vi "Startup.vi"(8 "error in (no error)":errorcluster, 11 "MyApp in":refnum<class "MyApp.lvclass">) -> (0 "error out":errorcluster, 3 "MyApp out":refnum<class "MyApp.lvclass">)   [LabVIEW 2012, in "MyApp.lvlib" / "MyApp.lvclass"]
uses:
  MyApp.lvclass
  HGF_DataAnalyzer/Wfm_Amplitude/Wfm_Amplitude.lvclass
  HGF_DataAnalyzer/Wfm_PulseMeasurement/Wfm_PulseMeasurement.lvclass
  HGF_DataAnalyzer/WfmAnalysator/WfmAnalysator.lvclass
  HGF_LVC/HGF_ApplicationBaseClasses/HGF_Application/HGF_Application.lvclass
  MyApp.lvclass/MyApp.ctl
  HGF_LVC/HGF_BaseClasses/HGF_Composite/HGF_Composite.lvclass
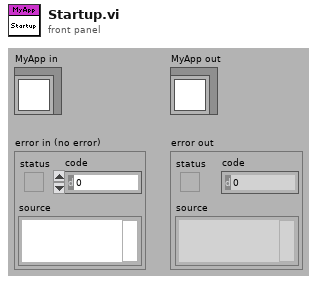
[diagram p1: front panel]
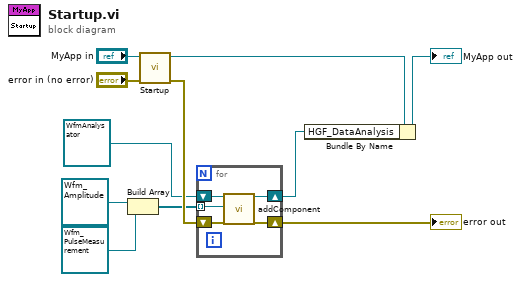
[diagram p0: block diagram]
diagram:
  n1 = Build Array(refnum<class "Wfm_Amplitude.lvclass"> refnum ("MyApp.lvlib:Wfm_Amplitude.lvclass"), refnum<class "Wfm_PulseMeasurement.lvclass"> refnum ("MyApp.lvlib:Wfm_PulseMeasurement.lvclass")) -> (w5:refnum<class "WfmAnalysator.lvclass">[])
  n2 = call-parent "Startup.vi"("error in (no error)"="error in (no error)", "HGF_Application in"="MyApp in") -> ("error out"=w8:errorcluster, "HGF_Application out"=w11:refnum<class "MyApp.lvclass">)  [unwired: 8 in]
  n3 = for {
    shift-right: [w15] -> w3
    shift-left: refnum<class "WfmAnalysator.lvclass"> refnum ("MyApp.lvlib:WfmAnalysator.lvclass") -> [w16]
    tunnel: w5 -> [w13] mode=indexing
    shift-right: [w12] -> w2
    shift-left: w8 -> [w14]
    n4 = call "addComponent.vi"("HGF_Composite"=w16, "HGF_Component"=w13, "error in (no error)"=w14) -> ("dup HGF_Composite"=w15:refnum<class "WfmAnalysator.lvclass">, "error out"=w12:errorcluster)  [unwired: 15 in]
  }
  "error out" <- w2
  n5 = Bundle By Name(cluster=w11, "HGF_DataAnalysis"=w3) -> (→"MyApp out":refnum<class "MyApp.lvclass">)
